vi "Decode Message.vi"(8 "Error In":errorcluster, 11 "Image 2 Path in":path) -> (0 "Error Out":errorcluster, 3 "Decoded Message":string)   [LabVIEW 2020]
uses:
  Image Comparison/Image Comparison.lvclass
panel:
  out "length":i32
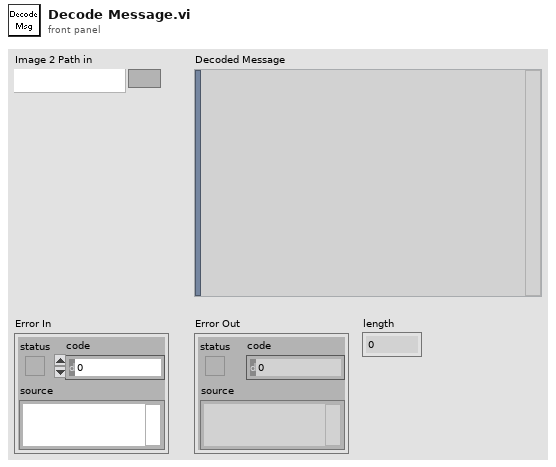
[diagram p1: front panel]
types:
  T1 = typedef "imagedata.ctl" = cluster{"image type":i32, "image depth":i32, "image":u8[], "mask":u8[], "colors":u32[], "Rectangle":cluster{"left":i16, "top":i16, "right":i16, "bottom":i16}}
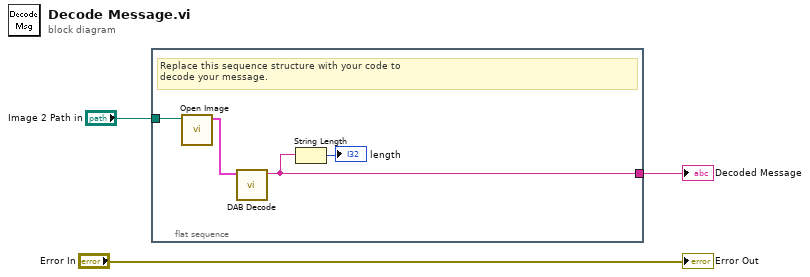
[diagram p0: block diagram]
diagram:
  n1 = flat-sequence {
    tunnel: [w5] -> w2
    tunnel: "Image 2 Path in" -> [w7]
    frame #0 {
      # "Replace this sequence structure with your code to \ndecode your message."
      n2 = call "Open Image.vi"("Image"=w7) -> ("image data"=w6:T1)  [unwired: 9 in, 1 out]
      n3 = call "DAB Decode.vi"("image data"=w6) -> ("Message"=w5:string)  [unwired: 10 in]
      n4 = String Length(string=w5) -> (length=→"length":i32)
    }
  }
  "Error Out" <- "Error In"
  "Decoded Message" <- w2
